vi "Set Logging.vi"(8 "error in":errorcluster, 11 "log?":bool) -> (0 "error out":errorcluster)   [LabVIEW 2017, in "myPAM.lvlib"]
uses:
  myPAM.lvlib
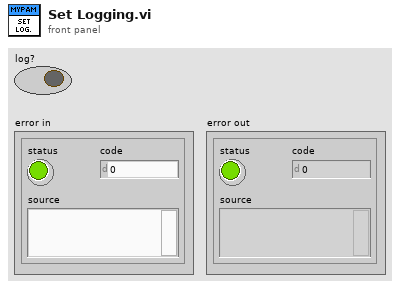
[diagram p1: front panel]
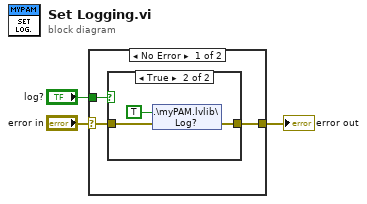
[diagram p0: block diagram]
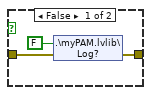
[diagram p2: hidden frame]
diagram:
  n1 = case shown="No Error" "error in" {
    selector: "error in" -> [w6 w13]
    tunnel: [w5 w13] -> w3
    tunnel: "log?" -> [w4 _]
    frame No Error {
      n2 = case shown="True" w4 {
        tunnel: w6 -> [w9 w12]
        tunnel: [w7 w11] -> w5
        frame False {
          n3 = shared-variable ".\\myPAM.lvlib\\Log?"(FALSE ("Log?"), error in=w9) -> (error out=w7:errorcluster)
        }
        frame True {
          n4 = shared-variable ".\\myPAM.lvlib\\Log?"(TRUE ("Log?"), error in=w12) -> (error out=w11:errorcluster)
        }
      }
    }
    frame Error {
    }
  }
  "error out" <- w3
